vi "ConfigureVelocityControllerWithObserver.vi"(0 "axis in":cluster{"keyHandle":u32, "nodeId":u16}={"keyHandle"=0, "nodeId"=1}, 5 "velocity gains":cluster{"p-Gain":u64, "i-Gain":u64}, 7 "feed forward gains":T2, 9 "observer gains":T1, 11 "error in (no error)":errorcluster) -> (4 "axis out":cluster{"keyHandle":u32, "nodeId":u16}={"keyHandle"=0, "nodeId"=1}, 15 "error out":errorcluster)   [LabVIEW 2017, in "maxonEPOS.lvlib"]
doc: "<B>ConfigureVelocityRegulator</B> writes the velocity regulation gain parameters to the device."
uses:
  Examples/maxonEPOS.lvlib
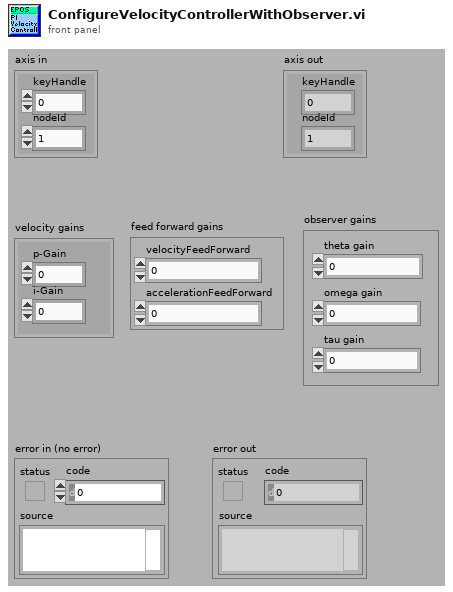
[diagram p1: front panel]
types:
  T1 = cluster{"theta gain":u64, "omega gain":u64, "tau gain":u64}
  T2 = cluster{"velocityFeedForward":u64, "accelerationFeedForward":u64}
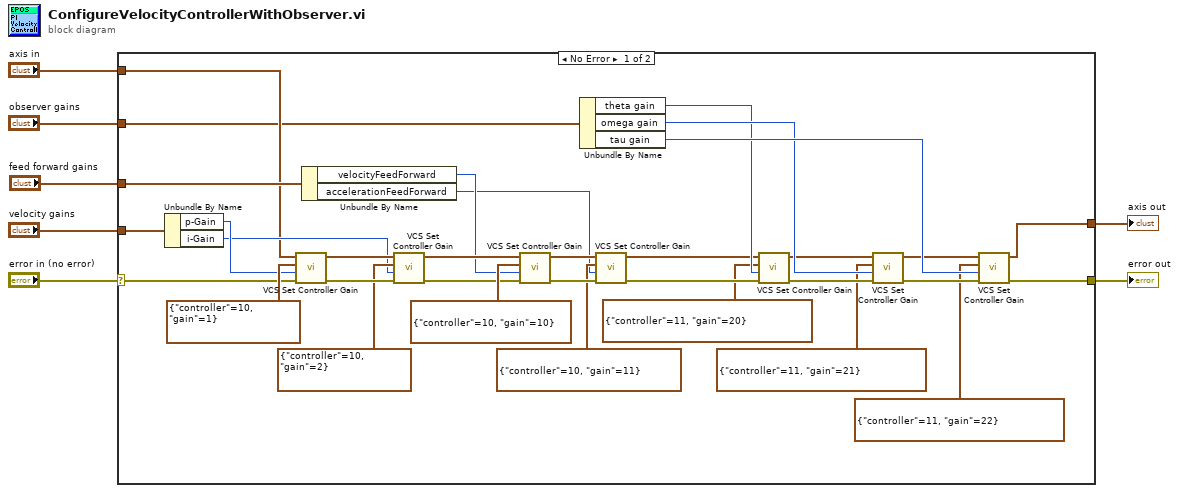
[diagram p0: block diagram]
diagram:
  n1 = case shown="No Error" "error in (no error)" {
    selector: "error in (no error)" -> [w30 w42]
    tunnel: [w11 w42] -> w6
    tunnel: [w15 w41] -> w5
    tunnel: "axis in" -> [w23 w41]
    tunnel: "velocity gains" -> [w29 _]
    tunnel: "feed forward gains" -> [w26 _]
    tunnel: "observer gains" -> [w22 _]
    frame No Error {
      n2 = Unbundle By Name(w29) -> ("p-Gain"=w28:u64, "i-Gain"=w27:u64)
      n3 = call "VCS Set Controller Gain.vi"("error in (no error)"=w30, "value"=w28, "controller gain"=cluster{"controller":u16, "gain":u16} {"controller"=10, "gain"=1}, "axis in"=w23) -> ("error out"=w40:errorcluster, "axis out"=w37:cluster{"keyHandle":u32, "nodeId":u16})  [unwired: 6 in]
      n4 = Unbundle By Name(w26) -> ("velocityFeedForward"=w25:u64, "accelerationFeedForward"=w24:u64)
      n5 = call "VCS Set Controller Gain.vi"("error in (no error)"=w40, "value"=w27, "controller gain"=cluster{"controller":u16, "gain":u16} {"controller"=10, "gain"=2}, "axis in"=w37) -> ("error out"=w32:errorcluster, "axis out"=w31:cluster{"keyHandle":u32, "nodeId":u16})  [unwired: 6 in]
      n6 = call "VCS Set Controller Gain.vi"("error in (no error)"=w32, "value"=w25, "controller gain"=cluster{"controller":u16, "gain":u16} {"controller"=10, "gain"=10}, "axis in"=w31) -> ("error out"=w39:errorcluster, "axis out"=w38:cluster{"keyHandle":u32, "nodeId":u16})  [unwired: 6 in]
      n7 = Unbundle By Name(w22) -> ("theta gain"=w19:u64, "omega gain"=w20:u64, "tau gain"=w21:u64)
      n8 = call "VCS Set Controller Gain.vi"("error in (no error)"=w39, "value"=w24, "controller gain"=cluster{"controller":u16, "gain":u16} {"controller"=10, "gain"=11}, "axis in"=w38) -> ("error out"=w14:errorcluster, "axis out"=w18:cluster{"keyHandle":u32, "nodeId":u16})  [unwired: 6 in]
      n9 = call "VCS Set Controller Gain.vi"("error in (no error)"=w14, "value"=w19, "controller gain"=cluster{"controller":u16, "gain":u16} {"controller"=11, "gain"=20}, "axis in"=w18) -> ("error out"=w13:errorcluster, "axis out"=w17:cluster{"keyHandle":u32, "nodeId":u16})  [unwired: 6 in]
      n10 = call "VCS Set Controller Gain.vi"("error in (no error)"=w13, "value"=w20, "controller gain"=cluster{"controller":u16, "gain":u16} {"controller"=11, "gain"=21}, "axis in"=w17) -> ("error out"=w12:errorcluster, "axis out"=w16:cluster{"keyHandle":u32, "nodeId":u16})  [unwired: 6 in]
      n11 = call "VCS Set Controller Gain.vi"("error in (no error)"=w12, "value"=w21, "controller gain"=cluster{"controller":u16, "gain":u16} {"controller"=11, "gain"=22}, "axis in"=w16) -> ("error out"=w11:errorcluster, "axis out"=w15:cluster{"keyHandle":u32, "nodeId":u16})  [unwired: 6 in]
    }
    frame Error {
    }
  }
  "error out" <- w6
  "axis out" <- w5
